vi "Read Digital Port.vi"(8 "error in (no error)":errorcluster, 11 "Abstract DMM in":refnum<class "DMM Instrument.lvclass">) -> (0 "error out":errorcluster, 2 "DIs":bool[](array[boolean]), 3 "Abstract DMM out":refnum<class "DMM Instrument.lvclass">)   [LabVIEW 2025, in "DMM.lvlib" / "DMM Instrument.lvclass"]
uses:
  DMM Instrument.lvclass
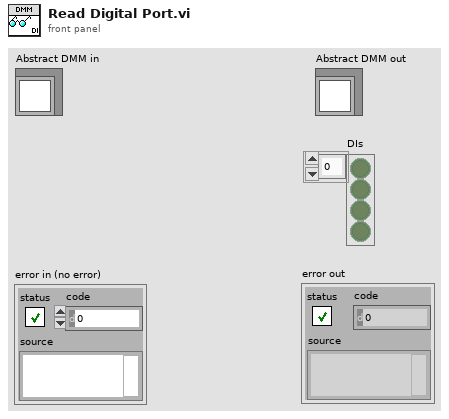
[diagram p1: front panel]
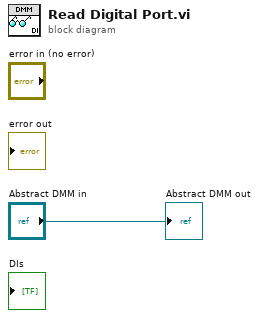
[diagram p0: block diagram]
diagram:
  "Abstract DMM out" <- "Abstract DMM in"
